vi "rspvtd_Configuration Data.vi"(8 "error in":errorcluster, 11 "Data in":variant) -> (0 "error out":errorcluster, 3 "Data out":T1={"Config Data"={"DS First Launch"=FALSE, "LogBaseFolder"=path "", "Live Logging"=FALSE, "Server Port"=0, "Max Number ML Rows"=0, "AM.WinBounds"={"Left"=0, "Top"=0, "Right"=0, "Bottom"=0}, "AM.FP.State"=enum."Invalid", "AM.Monitor"=0, "AM.Column Widths"=[], "ML.Visible Columns"=[], "ML.Splitter Position"=0, "ML.Column Widths"=[], "ML.WinBounds"={"Left"=0, "Top"=0, "Right"=0, "Bottom"=0}, "ML.FP.State"=enum."Invalid", "ML.Monitor"=0}})   [LabVIEW 2017, in "Settings.lvclass"]
doc: "This VI converts variant data contained in the associated <b>Public API Response</b> message to its correct data type.\n---"
uses:
  Settings.lvclass
  rsp_Configuration Data.ctl
  Config Data.ctl
  <vilib>/Utility/miscctls.llb/LVRectTypeDef.ctl
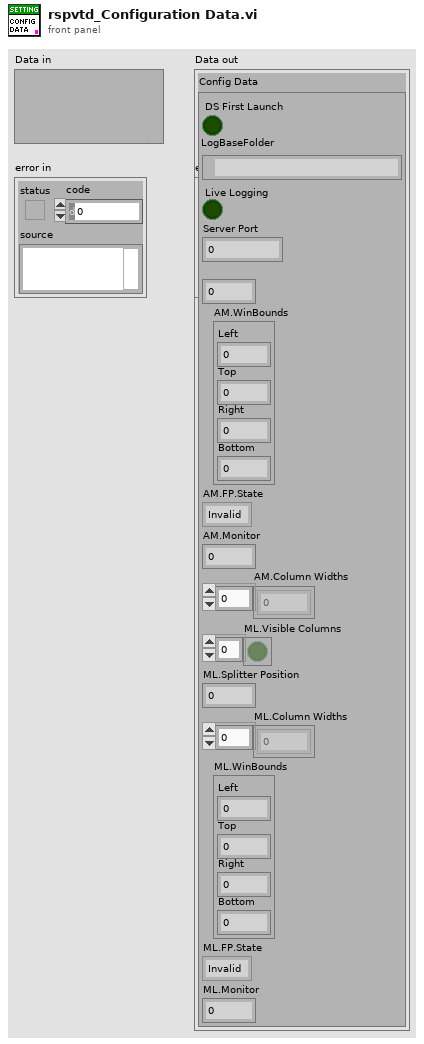
[diagram p1: front panel]
types:
  T1 = typedef "Settings.lvclass/rsp_Configuration Data.ctl" = cluster{"Config Data":T2}
  T2 = typedef "Settings.lvclass/Config Data.ctl" = cluster{"DS First Launch":bool, "LogBaseFolder":path, "Live Logging":bool, "Server Port":u16, "Max Number ML Rows":i32, "AM.WinBounds":T3, "AM.FP.State":enum32{"Invalid", "Standard", "Closed", "Hidden", "Minimized", "Maximized"}, "AM.Monitor":u16, "AM.Column Widths":u32[], "ML.Visible Columns":bool[], "ML.Splitter Position":i32, "ML.Column Widths":u32[], "ML.WinBounds":T3, "ML.FP.State":enum32{"Invalid", "Standard", "Closed", "Hidden", "Minimized", "Maximized"}, "ML.Monitor":u16}
  T3 = typedef "LVRectTypeDef.ctl" = cluster{"Left":i16, "Top":i16, "Right":i16, "Bottom":i16}
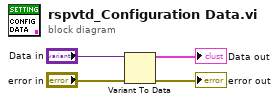
[diagram p0: block diagram]
diagram:
  n1 = Variant To Data(error in="error in", Variant="Data in") -> (data=→"Data out":T1, error out=→"error out":errorcluster)  [unwired: 1 in]
